vi "H5Pset_fill_time.vi"(6 "error in (no error)":errorcluster, 8 "Fill Time":T1 items=["H5D_FILL_TIME_ERROR"=-1, "H5D_FILL_TIME_ALLOC"=0, "H5D_FILL_TIME_NEVER"=1, "H5D_FILL_TIME_IFSET"=2], 9 "HDF5 Property Ref":T2) -> (0 "error out":errorcluster, 3 "HDF5 Ref out":T2)   [LabVIEW 2017]
doc: "Sets the time when fill values are written to a dataset."
uses:
  <vilib>/UPVI/lvhdf5/library.llb/HDF5 Ref.ctl
  <vilib>/UPVI/lvhdf5/property.llb/H5D_fill_time_t.ctl
  <vilib>/UPVI/lvhdf5/property.llb/H5D_layout_t.ctl
  <vilib>/UPVI/lvhdf5/hdf5.dll
panel:
  # "LVHDF5 Toolkit\nCopyright (c) 2005-2013 by Jason D. Sommerville\nCopyright (c) 2014 by UPVI, LLC.\n\nThis use and distribution of this file is governed by the terms found in \nLICENSE.txt distributed with this toolkit and installed at\n <user.lib>\\_lvhdf5\\LICENSE.txt"
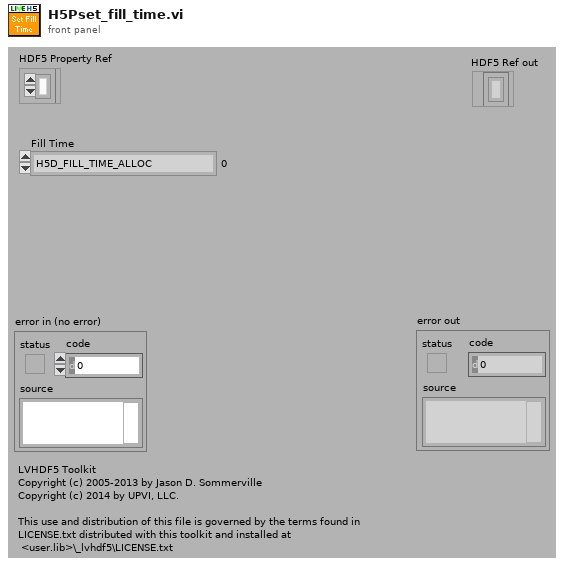
[diagram p1: front panel]
types:
  T1 = typedef "H5D_fill_time_t.ctl" = i32
  T2 = typedef "HDF5 Ref.ctl" = refnum<k1>
  T3 = typedef "H5D_layout_t.ctl" = i32
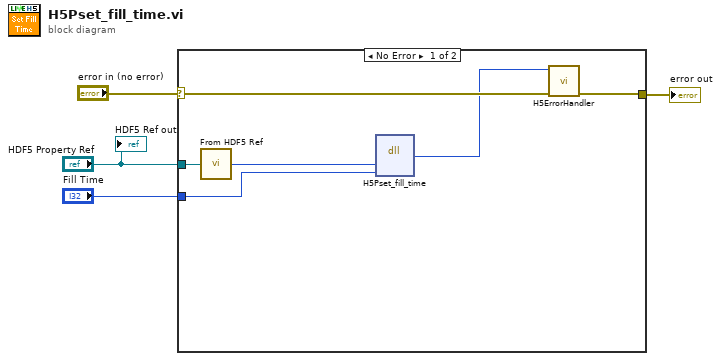
[diagram p0: block diagram]
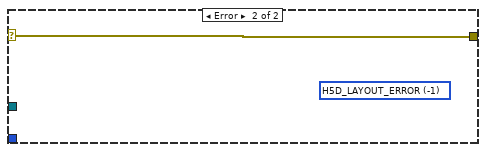
[diagram p2: hidden frame]
diagram:
  n1 = case shown="No Error" "error in (no error)" {
    selector: "error in (no error)" -> [w10 w11]
    tunnel: [w9 w11] -> w3
    tunnel: "HDF5 Property Ref" -> [w8 _]
    tunnel: "Fill Time" -> [w5 _]
    frame No Error {
      n2 = call <vilib>:"From HDF5 Ref.vi"("HDF5 Ref"=w8) -> ("I32"=w7:i32)
      n3 = dll-call lib="C:/Program Files/National Instruments/LabVIEW 2017/vi.lib/UPVI/lvhdf5/hdf5.dll" fn="H5Pset_fill_time"("plist_id"=w7, "fill_time"=w5) -> (w6:i32)  [unwired: 5 in, 2 out]
      n4 = call <vilib>:"H5ErrorHandler.vi"("error in (no error)"=w10, "herr_t"=w6) -> ("error out"=w9:errorcluster)  [unwired: 3 in, 4 out]
    }
    frame Error {
      (unwired) T3 -1 items=["H5D_LAYOUT_ERROR"=-1, "H5D_COMPACT"=0, "H5D_CONTIGUOUS"=1, "H5D_CHUNKED"=2] ("Layout")
    }
  }
  "error out" <- w3
  "HDF5 Ref out" <- "HDF5 Property Ref"
